vi "Init.vi"(4 "Rename":string, 6 "Name":string, 9 "Project:Active Project":refnum<vi>) -> (3 "Script out":refnum<class "_Rename.lvclass">)   [LabVIEW 2021, in "_Rename.lvlib" / "_Rename.lvclass"]
uses:
  _Rename.lvclass
  _Rename.lvclass/_Rename.ctl
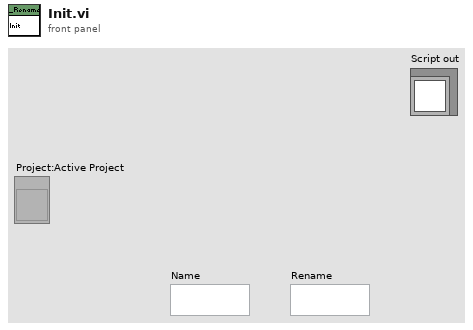
[diagram p1: front panel]
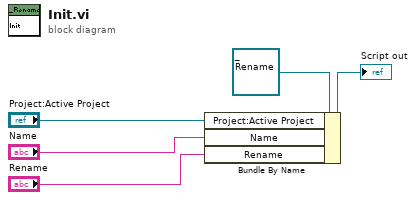
[diagram p0: block diagram]
diagram:
  n1 = Bundle By Name(cluster=refnum<class "_Rename.lvclass"> refnum ("Script out"), "Project:Active Project"="Project:Active Project", "Name"="Name", "Rename"="Rename") -> (→"Script out":refnum<class "_Rename.lvclass">)
